vi "LVClass_ComputePhaseSet SetModalFilter.vi"(0 "ComputePhaseSet in":refnum<class "ComputePhaseSet.lvclass">, 5 "polynomial_number_to_filter":u32[](array[numeric]), 11 "error in (no error)":errorcluster) -> (4 "ComputePhaseSet out":refnum<class "ComputePhaseSet.lvclass">, 15 "error out":errorcluster)   [LabVIEW 2020, in "ComputePhaseSet.lvclass"]
doc: "Set filter for phase reconstruction from modal decomposition. The filter is\ndefined by the indices of polynomials that must be filtered.\n\n<B>ComputePhaseSetIn</B> : ComputePhaseSet object.\n<B>ComputePhaseSetOut</B> : ComputePhaseSet object.\n<B>nb_coeffs_to_filter</B> : Number of the coefficients to filter in the polynomial base.\n<B>coeffs_to_filter</B> : List of indices of the coefficients to filter in the polynomial base."
uses:
  ComputePhaseSet.lvclass
  ComputePhaseSet.lvclass/ComputePhaseSet.ctl
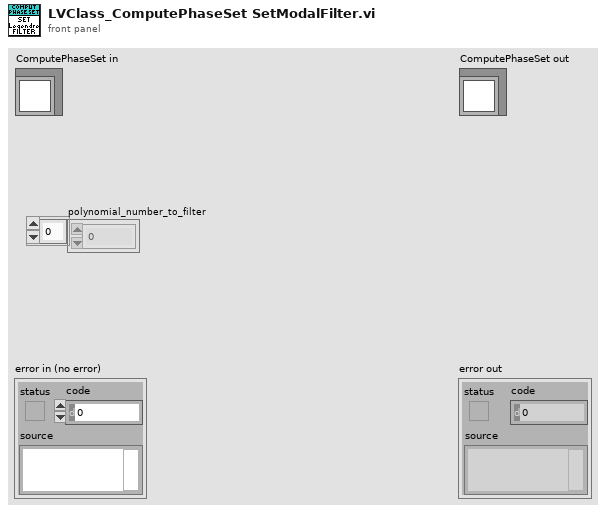
[diagram p1: front panel]
types:
  T1 = typedef "ClassID.ctl" = i64
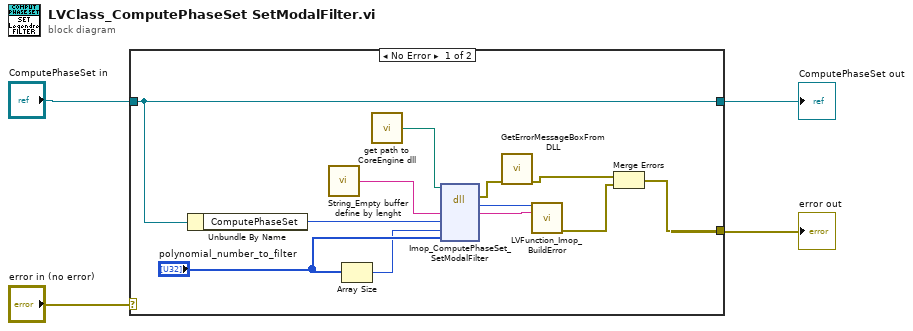
[diagram p0: block diagram]
diagram:
  n1 = case shown="No Error" "error in (no error)" {
    selector: "error in (no error)" -> [_ w18]
    tunnel: [w5 w18] -> w1
    tunnel: [w9 w17] -> w3
    tunnel: "ComputePhaseSet in" -> [w9 w17]
    frame No Error {
      n2 = Unbundle By Name(w9) -> ("ComputePhaseSet"=w8:T1)
      n3 = call "String_Empty buffer define by lenght.vi"() -> ("Empty buffer"=w14:string)  [unwired: 1 in]
      n4 = Array Size(array="polynomial_number_to_filter") -> (size(s)=w10:i32)
      n5 = call "get path to CoreEngine dll.vi"() -> ("path to wavekit library"=w13:path)  [unwired: 14 in, 1 out]
      n6 = dll-call lib="D:/2_trunk/temp_core_engine/DLLs/ImopEngine4_vc100.dll" fn="Imop_ComputePhaseSet_SetModalFilter"(path in=w13, "message"=w14, "objet"=w8, "nb_to_filter"=w10, "polynomial_number_to_filter"="polynomial_number_to_filter") -> (error out=w12:errorcluster, "return type"=w16:i32, "message"=w15:string)  [unwired: 5 in, 1 out]
      n7 = call "GetErrorMessageBoxFromDLL.vi"("error IN"=w12) -> ("error OUT"=w7:errorcluster)  [unwired: 10 in]
      n8 = call "LVFunction_Imop_BuildError.vi"("code"=w16, "String to Prepend to source (\"\")"=w15) -> ("error out"=w6:errorcluster)  [unwired: 13 in]
      n9 = Merge Errors(w7, w6) -> (w5:errorcluster)
    }
    frame Error {
    }
  }
  "error out" <- w1
  "ComputePhaseSet out" <- w3
